vi "FlatToRichnidevice_grpc_EnumerateDevicesResponse.vi"(5 "OutputClusterType":T1, 11 "InputCluster":T3) -> (3 "OutputCluster":T1)   [LabVIEW 2021, in "NI DAQmx_server.lvlib"]
uses:
  NI DAQmx_server.lvlib
  nidevice_grpc_EnumerateDevicesResponse_Flat.ctl
  nidevice_grpc_DeviceProperties_Flat.ctl
  nidevice_grpc_EnumerateDevicesResponse.ctl
  nidevice_grpc_DeviceProperties.ctl
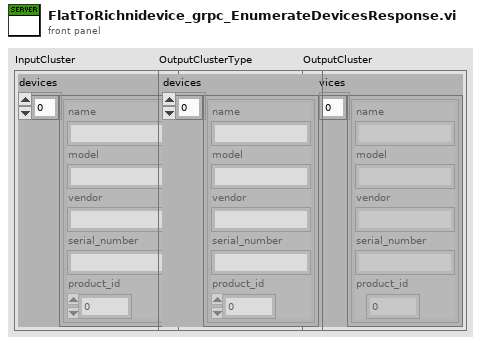
[diagram p1: front panel]
types:
  T1 = typedef "NI DAQmx_server.lvlib/nidevice_grpc_EnumerateDevicesResponse.ctl" = cluster{"devices":T2[]}
  T2 = typedef "NI DAQmx_server.lvlib/nidevice_grpc_DeviceProperties.ctl" = cluster{"name":string, "model":string, "vendor":string, "serial_number":string, "product_id":u32}
  T3 = typedef "NI DAQmx_server.lvlib/nidevice_grpc_EnumerateDevicesResponse_Flat.ctl" = cluster{"devices":T4[]}
  T4 = typedef "NI DAQmx_server.lvlib/nidevice_grpc_DeviceProperties_Flat.ctl" = cluster{"name":string, "model":string, "vendor":string, "serial_number":string, "product_id":u32}
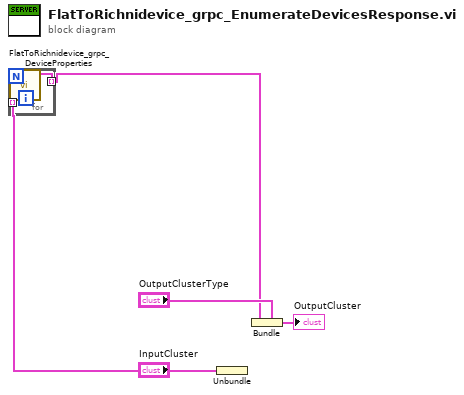
[diagram p0: block diagram]
diagram:
  n1 = Unbundle "Unbundle"("InputCluster") -> ("devices"=w2:T4[])
  n2 = for {
    tunnel: w2 -> [w7] mode=indexing
    tunnel: [w6] -> w1 mode=indexing
    n3 = call "FlatToRichnidevice_grpc_DeviceProperties.vi"("InputCluster"=w7) -> ("OutputCluster"=w6:T2)  [unwired: 10 in]
  }
  n4 = Bundle "Bundle"(cluster="OutputClusterType", "devices"=w1) -> (→"OutputCluster":T1)
